vi "endEventToString.vi"(8 "error in (no error)":errorcluster, 11 "RampToneUp in":refnum<class "RampToneUp.lvclass">) -> (0 "error out":errorcluster, 3 "RampToneUp out":refnum<class "RampToneUp.lvclass">)   [LabVIEW 2011, in "Tools.lvlib" / "Scripting.lvlib" / "RampToneUp.lvclass"]
uses:
  RampToneUp.lvclass
  SingleTone/SingleTone.lvclass
  RampTone/RampTone.lvclass
panel:
  out "eventStringArray":string[](array[string])
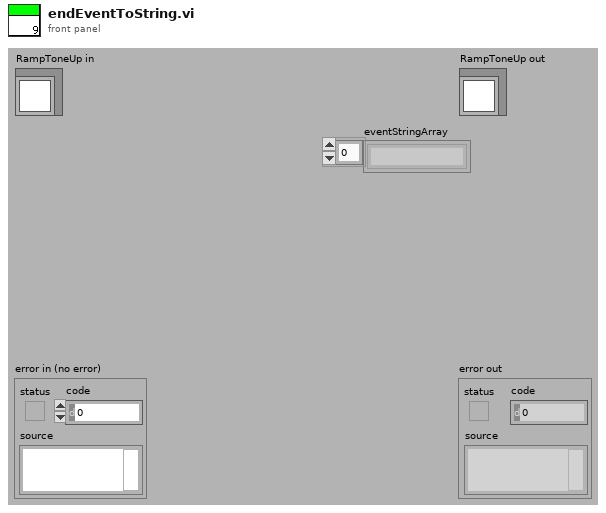
[diagram p1: front panel]
types:
  T1 = cluster{"rampTime":dbl, "timeStep":dbl, "dataValueStep":dbl}
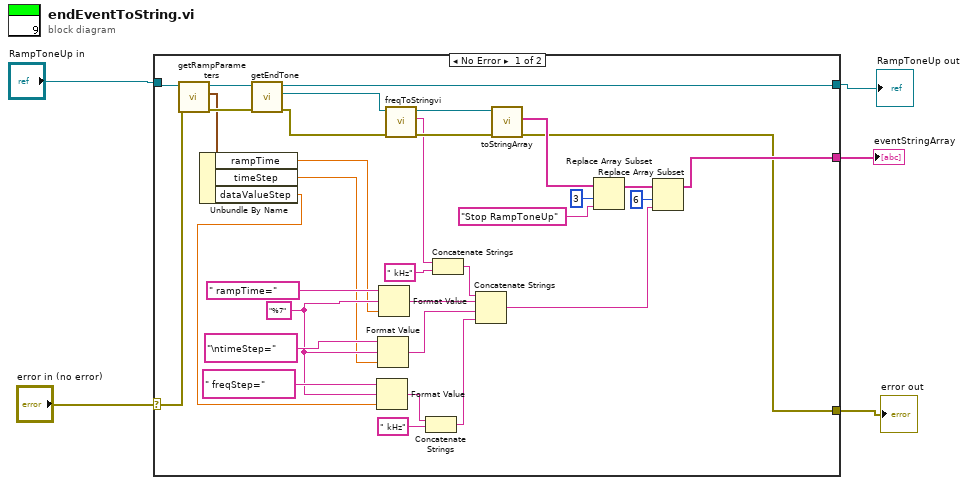
[diagram p0: block diagram]
diagram:
  n1 = case shown="No Error" "error in (no error)" {
    selector: "error in (no error)" -> [w10 w39]
    tunnel: [w20 w39] -> w3
    tunnel: [w25 _] -> w2
    tunnel: "RampToneUp in" -> [w16 w40]
    tunnel: [w14 w40] -> w4
    frame No Error {
      w24 = "%7"
      n2 = call "getRampParameters.vi"("error in (no error)"=w10, "RampTone in"=w16) -> ("error out"=w13:errorcluster, "RampParameters"=w9:T1, "RampTone out"=w15:refnum<class "RampToneUp.lvclass">)  [unwired: 7 in]
      n3 = Unbundle By Name(w9) -> ("rampTime"=w8:dbl, "timeStep"=w7:dbl, "dataValueStep"=w6:dbl)
      n4 = call-dynamic "getEndTone.vi"("error in (no error)"=w13, "RampTone.lvclass in"=w15) -> ("error out"=w12:errorcluster, "endTone.lvclass"=w11:refnum<class "SingleTone.lvclass">, "RampTone.lvclass out"=w14:refnum<class "RampToneUp.lvclass">)  [unwired: 7 in]
      n5 = Format Value(string ("")=" freqStep=", format string=w24, value (0)=w6) -> (output string=w28:string)
      n6 = Format Value(string ("")="\ntimeStep=", format string=w24, value (0)=w7) -> (output string=w30:string)
      n7 = Format Value(string ("")=" rampTime=", format string=w24, value (0)=w8) -> (output string=w31:string)
      n8 = call-dynamic "freqToStringvi.vi"("error in (no error)"=w12, "SingleTone in"=w11) -> ("error out"=w19:errorcluster, "frequency"=w17:string, "SingleTone out"=w18:refnum<class "SingleTone.lvclass">)  [unwired: 7 in]
      n9 = Concatenate Strings(w28, " kHz") -> (w26:string)
      n10 = Concatenate Strings(w17, " kHz") -> (w22:string)
      n11 = Concatenate Strings(w22, w31, w30, w26) -> (w29:string)
      n12 = call-dynamic "toStringArray.vi"("error in (no error)"=w19, "SingleTone in"=w18) -> ("error out"=w20:errorcluster, "eventStringArray"=w21:string[])  [unwired: 7 in, 1 out]
      n13 = Replace Array Subset(array=w21, new element="Stop RampToneUp", index=3) -> (w34:string[])
      n14 = Replace Array Subset(array=w34, new element=w29, index=6) -> (w25:string[])
    }
    frame Error {
    }
  }
  "error out" <- w3
  "RampToneUp out" <- w4
  "eventStringArray" <- w2
